vi "G#Object_GetOwner.vi"(0 "reference in":refnum<class "G#RemoteProxy.lvclass">, 5 "error in (no error)":errorcluster) -> (14 "reference out":refnum<class "G#RemoteProxy.lvclass">, 16 "owner":string, 19 "error out":errorcluster)   [LabVIEW 2017, in "G#RemoteProxy.lvclass"]
doc: "Returns the top-level owning VI name of the object."
uses:
  <vilib>/addons/_AddQ/G#Debugger/G#RemoteProxy/G#RemoteProxy.lvclass
  <vilib>/addons/_AddQ/G#Debugger/G#RemoteProxy/G#RemoteProxy.lvclass/G#RemoteProxy.ctl
  <vilib>/addons/_AddQ/G#Object/G#Object.lvclass
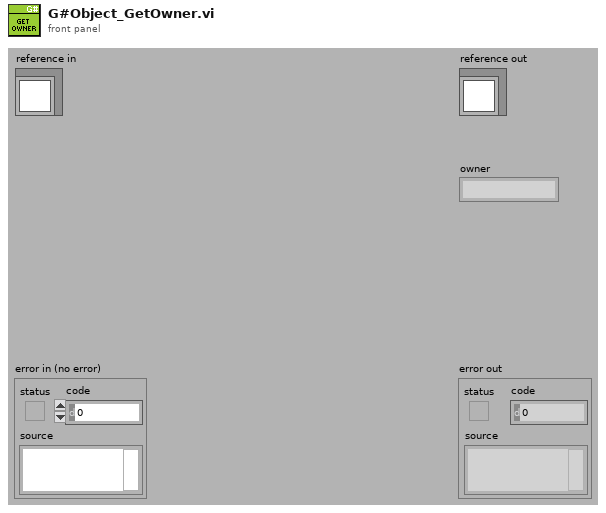
[diagram p1: front panel]
types:
  T1 = typedef "G#RemoteProxy.lvclass/ObjectAttributesProxy.ctl" = cluster{"class hierarchy":T2[], "class name":string, "lvlib hierarchy":string[], "full class name":string, "id":u32, "owner":string, "RemoteRef":refnum<class "G#Object.lvclass">, "object name":string, "attributes":variant[], "connection ID":refnum<k5>, "address":u32, "occurrence":refnum<k4>, "ProxyClassRef":refnum<class "G#RemoteProxy.lvclass">, "InMemory?":bool, "ToString":string}
  T2 = typedef "G#Object.lvclass/G#Object_ClassHierarchy.ctl" = cluster{"ClassName":string, "FullClassName":string, "ClassPath":path, "IsLeaf":bool}
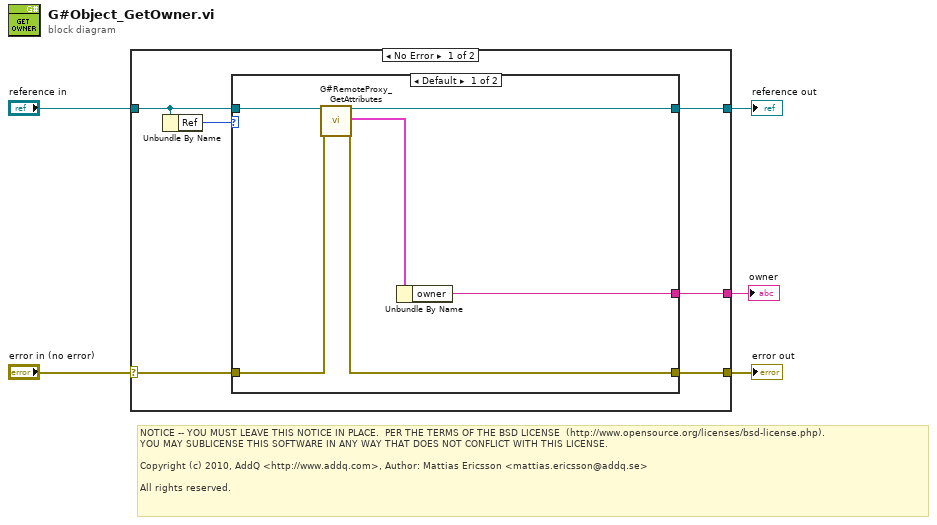
[diagram p0: block diagram]
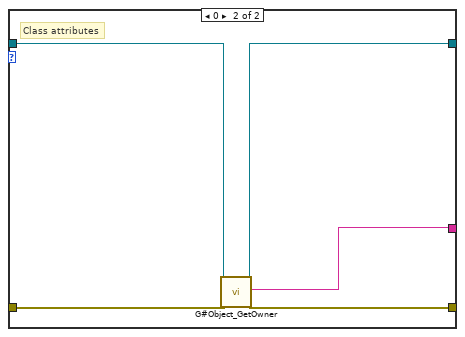
[diagram p2: hidden frame]
diagram:
  # "NOTICE -- YOU MUST LEAVE THIS NOTICE IN PLACE.  PER THE TERMS OF THE BSD LICENSE  (http://www.opensource.org/licenses/bsd-license.php).\nYOU MAY SUBLICENSE THIS SOFTWARE IN ANY WAY THAT DOES NOT CONFLICT WITH THIS LICENSE.\n\nCopyright (c) 2010, AddQ <http://www.addq.com>, Author: Mattias Ericsson <mattias.ericsson@addq.se>\n\nAll rights reserved."
  n1 = case shown="No Error" "error in (no error)" {
    selector: "error in (no error)" -> [w10 w24]
    tunnel: [w9 w24] -> w4
    tunnel: [w11 w23] -> w2
    tunnel: "reference in" -> [w7 w23]
    tunnel: [w8 _] -> w1
    frame No Error {
      n2 = Unbundle By Name(w7) -> ("Ref"=w6:u32)
      n3 = case shown="Default" w6 {
        tunnel: [w17 w21] -> w11
        tunnel: w10 -> [w16 w20]
        tunnel: [w15 w19] -> w9
        tunnel: [w12 w18] -> w8
        tunnel: w7 -> [w13 w22]
        frame Default {
          n4 = call <vilib>:"G#RemoteProxy_GetAttributes.vi"("reference in"=w13, "error in (no error)"=w16) -> ("reference out"=w17:refnum<class "G#RemoteProxy.lvclass">, "attributes"=w14:T1, "error out"=w15:errorcluster)  [unwired: 14 in, 1 out]
          n5 = Unbundle By Name(w14) -> ("owner"=w12:string)
        }
        frame 0 {
          # "Class attributes"
          n6 = call-parent "G#Object_GetOwner.vi"("reference in"=w22, "error in (no error)"=w20) -> ("reference out"=w21:refnum<class "G#RemoteProxy.lvclass">, "owner"=w18:string, "error out"=w19:errorcluster)  [unwired: 15 in]
        }
      }
    }
    frame Error {
    }
  }
  "error out" <- w4
  "reference out" <- w2
  "owner" <- w1
